vi "Der_W.vi"(1 "dA_l-1":T1, 2 "dZ_l":T1, 3 "m":dbl) -> (0 "dW_l":T1)   [LabVIEW 2016]
uses:
  <vilib>/Analysis/Matrix/Datatypes/RealMatrix.ctl
  <vilib>/Analysis/Matrix/Numeric/Multiply/Multiply - RM,RM.vi
  <vilib>/Analysis/Matrix/Numeric/Conversions/Matrix To Array - RM.vi
  <vilib>/Analysis/Matrix/Numeric/Conversions/Array To Matrix - RA2.vi
  <vilib>/Analysis/Matrix/NI_Matrix.lvlib
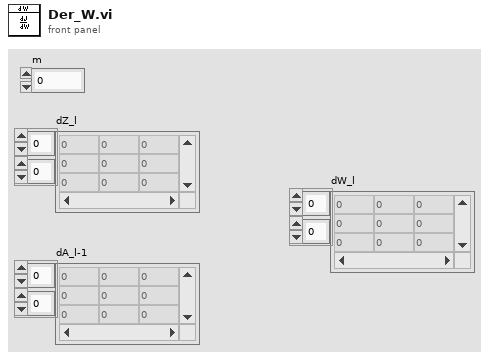
[diagram p1: front panel]
types:
  T1 = typedef "NI_Matrix.lvlib/RealMatrix.ctl" = dbl[][]
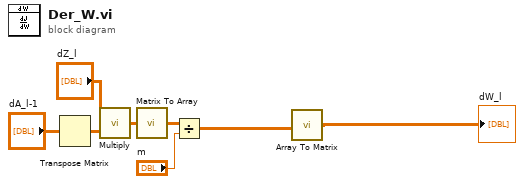
[diagram p0: block diagram]
diagram:
  n1 = Transpose Matrix(1:"dA_l-1") -> (0:w6:T1)
  n2 = call-poly <vilib>:"Multiply.vi"("Real Matrix B"=w6, "Real Matrix A"="dZ_l") -> ("A * B"=w5:T1)
  n3 = call-poly <vilib>:"Matrix To Array.vi"("Real Matrix"=w5) -> ("Real 2D Array"=w4:dbl[][])
  n4 = Divide(x=w4, y="m") -> (x/y=w2:dbl[][])
  n5 = call-poly <vilib>:"Array To Matrix.vi"("Real 2D Array"=w2) -> ("Real Matrix"=→"dW_l":T1)
